vi "labview_import.vi"() -> ()   [LabVIEW 2011]
uses:
  <vilib>/Platform/TimedLoop/XDataNode/timing_clust.ctl
  <vilib>/Platform/TimedLoop/XDataNode/nitl_modes.ctl
  <vilib>/Platform/TimedLoop/XDataNode/wakeup.ctl
  <vilib>/Platform/TimedLoop/XDataNode/XDataNode.xnode
  <vilib>/Easy HTTP Client/Easy HTTP.lvlib
  <vilib>/LVH/i3 JSON/i3-json.lvlib
  <vilib>/Platform/TimedLoop/XDataNode/XDNodeRunTimeDep.lvlib
panel:
  in  "Loop!":bool
  out "Cluster 3":T1 {"timestamp" format="%#.2f"; "temperature" scale=0.0..100.0}
  in  "Cluster":T1 {"temperature" scale=0.0..100.0}
  out "body":string
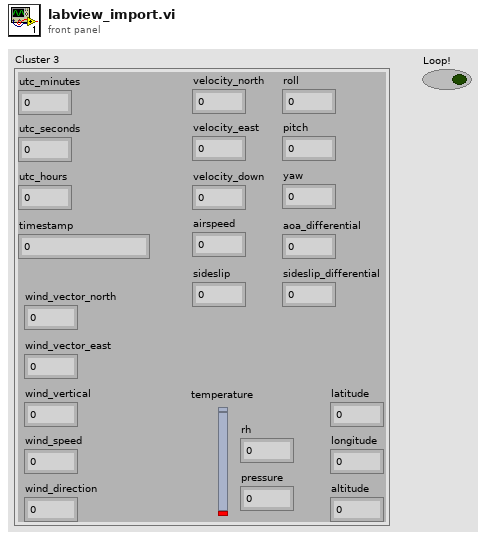
[diagram p1: front panel]
types:
  T1 = cluster{"utc_minutes":dbl, "utc_seconds":dbl, "utc_hours":dbl, "rh":dbl, "pressure":dbl, "wind_vector_north":dbl, "wind_vector_east":dbl, "wind_speed":dbl, "wind_direction":dbl, "latitude":dbl, "longitude":dbl, "altitude":dbl, "velocity_north":dbl, "velocity_east":dbl, "velocity_down":dbl, "roll":dbl, "pitch":dbl, "yaw":dbl, "airspeed":dbl, "wind_vertical":dbl, "sideslip":dbl, "aoa_differential":dbl, "sideslip_differential":dbl, "temperature":dbl, "timestamp":dbl}
  T2 = typedef "XDNodeRunTimeDep.lvlib/timing_clust.ctl" = cluster{"Expected End [f-1]":u64, "Actual End [f-1]":u64, "Finished Late? [f-1]":bool, "Expected End [i-1]":u64, "Actual End [i-1]":u64, "Finished Late? [i-1]":bool, "Expected Start [i]":u64, "Actual Start [i]":u64, "Expected Start [f]":u64, "Actual Start [f]":u64, "Source Name":string, "Structure Name":string, "Period":i64, "Deadline":i64, "Offset":i64, "Start":i64, "Priority":i32, "Timeout":i32, "Mode":T3, "Wakeup Reason":T4, "Error":errorcluster, "Source Type":string, "Secondary Source Type":string, "Global End Time":u64, "Global Start Time":u64, "Frame Duration":u64, "Iteration Duration":u64, "Assigned CPU":i32, "I/O Scan Engine Mode":u32}
  T3 = typedef "XDNodeRunTimeDep.lvlib/nitl_modes.ctl" = enum32{"No Change", "Process missed periods, maintain original phase", "Discard missed periods, maintain original phase", "Process missed periods, ignore original phase", "Discard missed periods, ignore original phase"}
  T4 = typedef "XDNodeRunTimeDep.lvlib/wakeup.ctl" = enum32{"Normal", "Aborted", "Asynchronous wakeup", "Timing source error", "Timed loop error", "Timeout"}
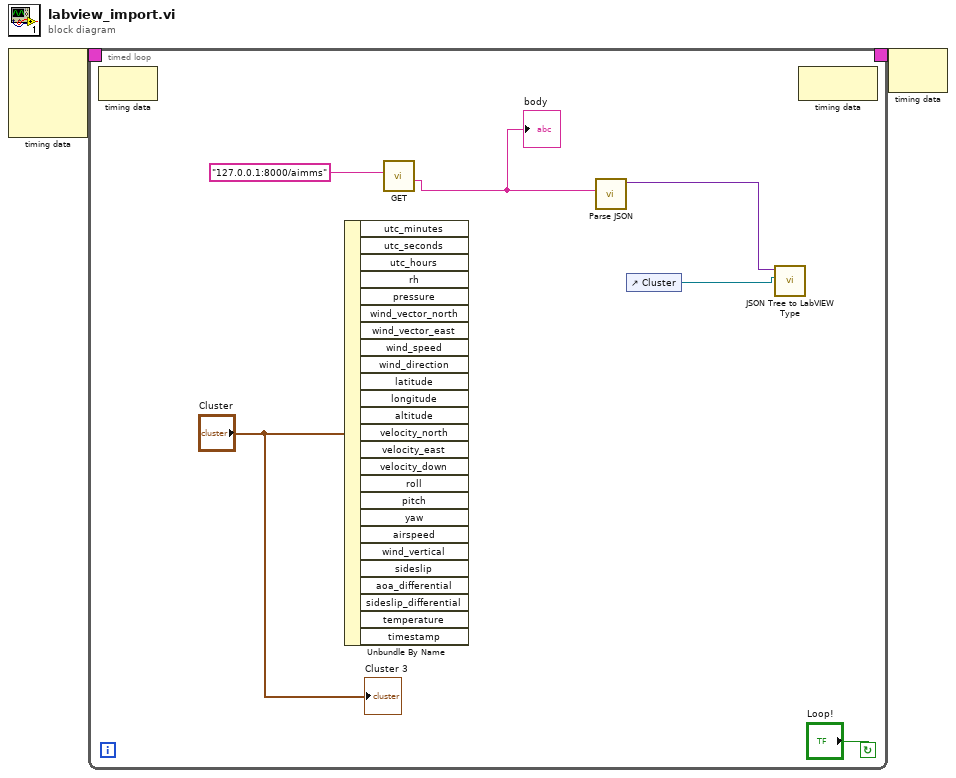
[diagram p0: block diagram]
diagram:
  n1 = node-c288() -> (w2:T2)  [unwired: 4 in]
  n2 = timed-loop {
    timing: w2 -> [_]
    timing-out: [_] -> w1
    stop <- "Loop!" continue-if-true
    n3 = node-c288() -> ()  [unwired: 1 in, 1 out]
    n4 = Unbundle By Name("Cluster") -> ()  [unwired: 25 out]
    n5 = call <vilib>:"GET.vi"("url"="127.0.0.1:8000/aimms") -> ("body"=w7:string)  [unwired: 6 in, 4 out]
    "body" <- w7
    n6 = call <vilib>:"Parse JSON.vi"("JSON String"=w7) -> ("JSON Tree"=w6:variant)  [unwired: 7 in, 3 out]
    n7 = control-ref of="Cluster"() -> (w5:refnum<vi>)
    n8 = call <vilib>:"JSON Tree to LabVIEW Type.vi"("Ctl Refnum"=w5, "JSON Tree In"=w6) -> ()  [unwired: 8 in, 2 out]
    n9 = node-c288() -> ()  [unwired: 1 in, 1 out]
    "Cluster 3" <- "Cluster"
  }
  n10 = node-c288(w1) -> ()  [unwired: 1 out]
